vi "写入内置参数.vi"(7 "量程参数读取":T3 {"阈值（高->低）" format="%#.6g"; "阈值（低->高）" format="%#.6g"; "下限" format="%#.6g"; "上限" format="%#.6g"}, 8 "error in (no error)":errorcluster, 9 "float":T2 {"偏心轮校准参数" format="%#.6g"}, 10 "外设配置":T1 {"是否存在液位检测板" items=["否", "是"]; "阀数量" items=["9通"=9, "12通"=12]; "泵类型" items=["TECAN", "润泽"]}, 11 "MB session in":refnum<class "MB_Master.lvclass">) -> (0 "error out":errorcluster, 3 "MB session out":refnum<class "MB_Master.lvclass">)   [LabVIEW 2016, in "斯坦道CODMn新电路板.lvlib"]
uses:
  <vilib>/Plasmionique/MB Master/MB_Master/MB_Master.lvclass
  <vilib>/Plasmionique/MB Master/MB_Master_Serial/MB_Master_Serial.lvclass
  D:/Program Files (x86)/National Instruments/LabVIEW 2016/vi.lib/Plasmionique/MB Master/MB_Master/MB_Master.lvclass
  <vilib>/Plasmionique/MB Master/MB Master.lvlib
panel:
  in  "VISA Resource":refnum<visa-resource-name>
  in  "引用选择":enum16{"MB引用", "自建引用"}(ring)
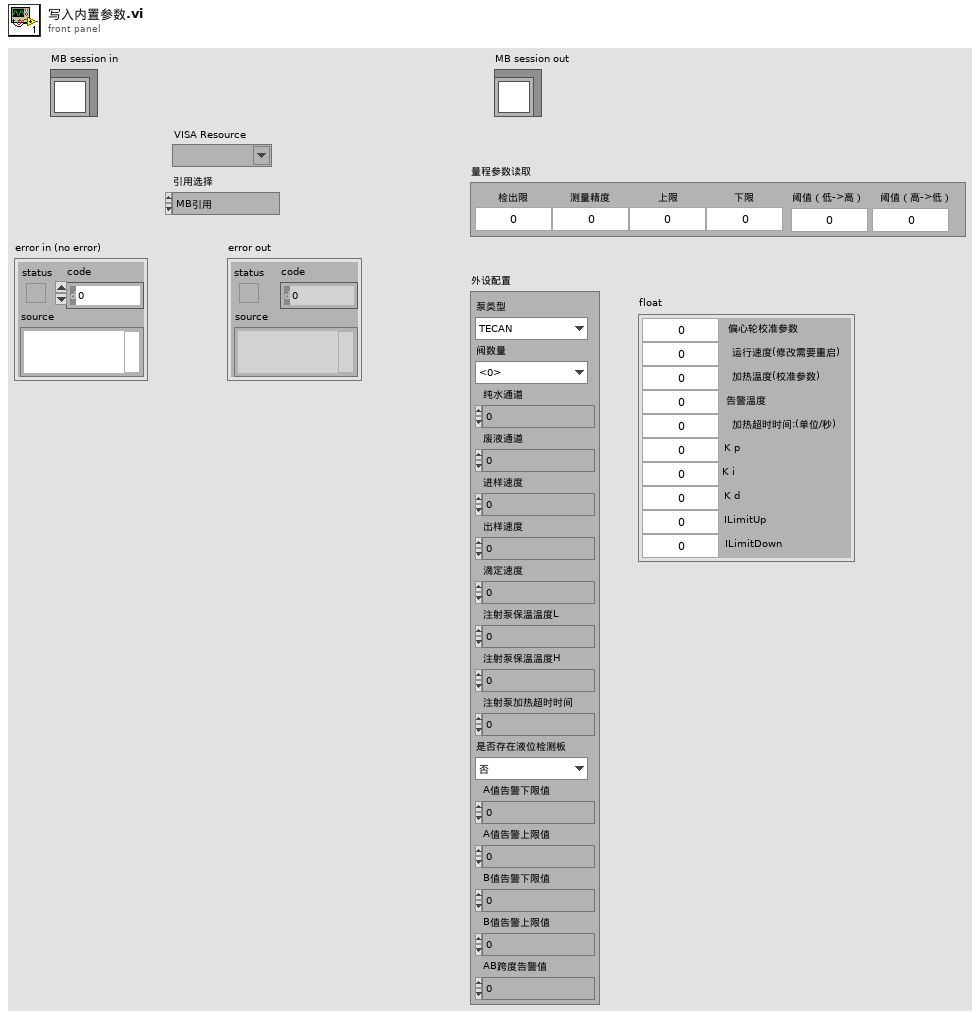
[diagram p1: front panel]
types:
  T1 = cluster{"泵类型":u8, "阀数量":u8, "纯水通道":u8, "废液通道":u8, "进样速度":u16, "出样速度":u16, "滴定速度":u16, "注射泵保温温度L":u8, "注射泵保温温度H":u8, "注射泵加热超时时间":u16, "是否存在液位检测板":u16, "A值告警下限值":u16, "A值告警上限值":u16, "B值告警下限值":u16, "B值告警上限值":u16, "AB跨度告警值":u16}
  T2 = cluster{"偏心轮校准参数":dbl, "运行速度(修改需要重启)":u16, "加热温度(校准参数) ":dbl, "告警温度":dbl, "加热超时时间:(单位/秒)":dbl, "K p":dbl, "K i":dbl, "K d":dbl, "ILimitUp":dbl, "ILimitDown":dbl}
  T3 = cluster{"检出限":dbl, "测量精度":dbl, "上限":dbl, "下限":dbl, "阈值（低->高）":dbl, "阈值（高->低）":dbl}
  T4 = cluster{"baud rate (bps)":u32, "stop bits":u16, "parity":u16, "flow control":u16, "timeout":u32, "retries":i32}
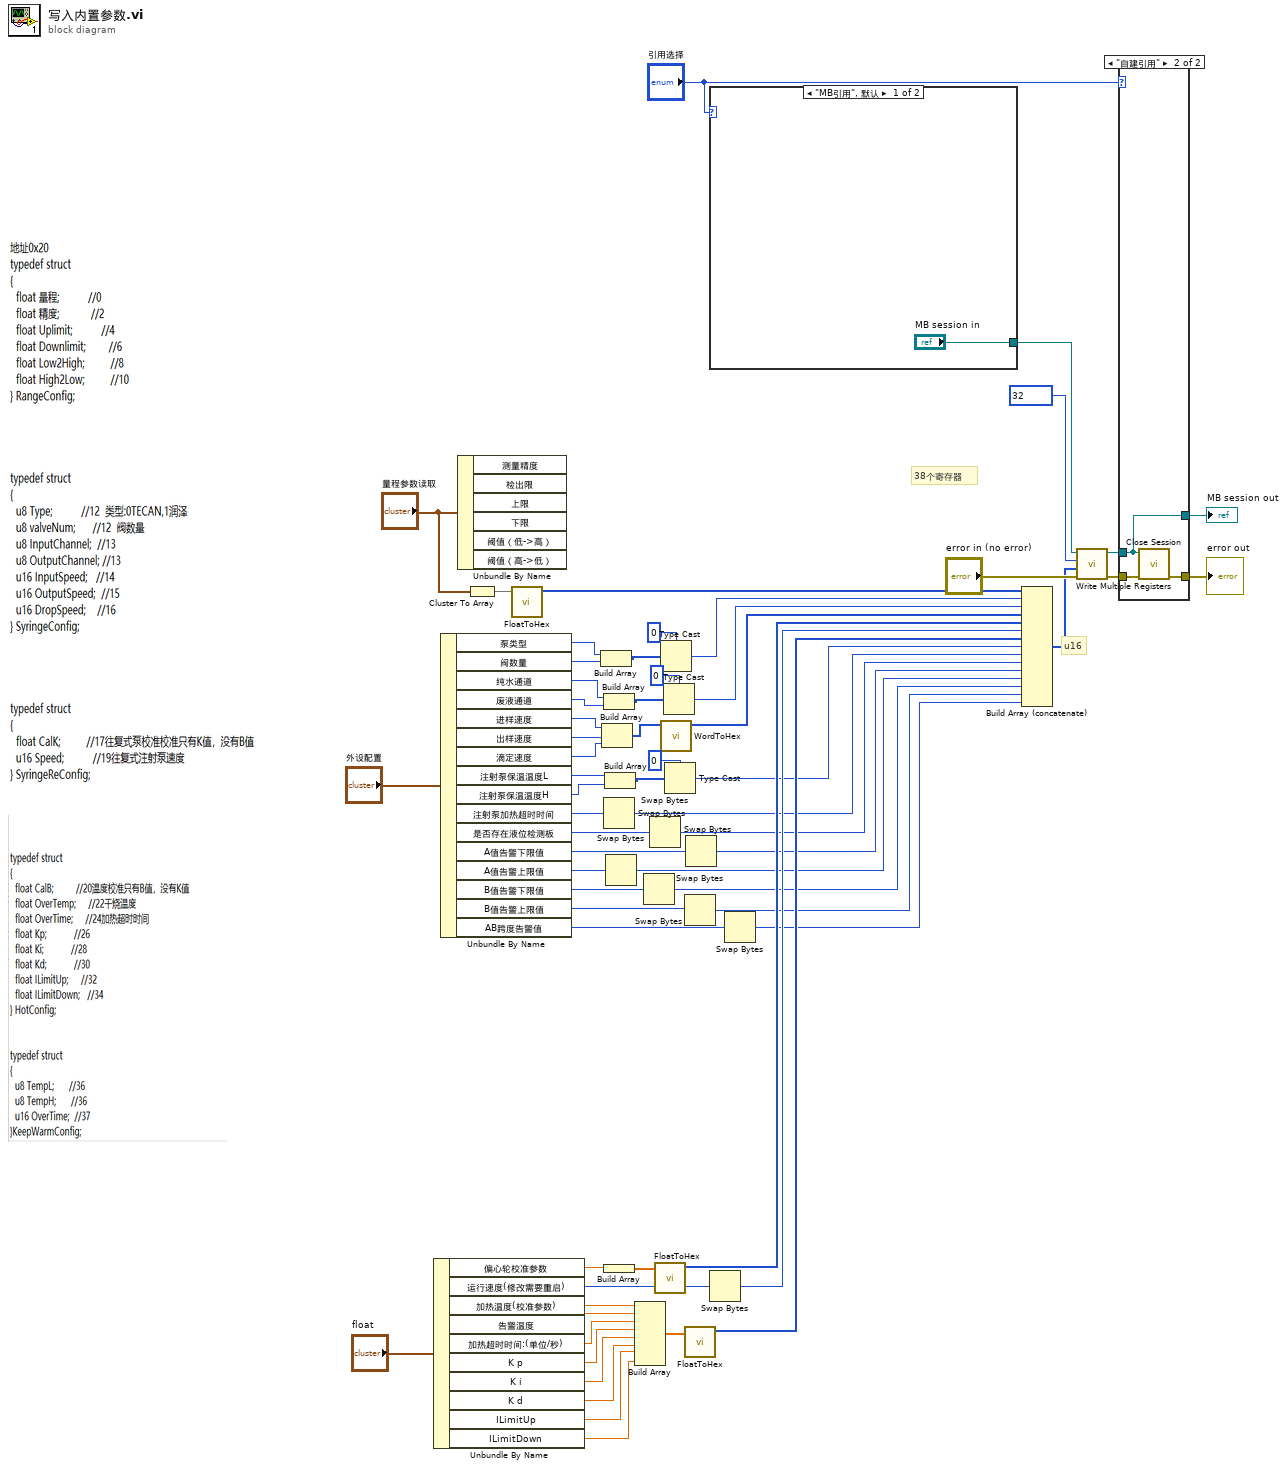
[diagram p0: block diagram]
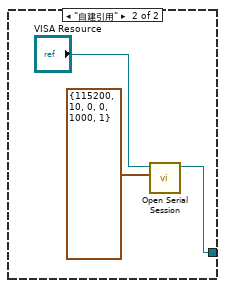
[diagram p3: hidden frame]
diagram:
  # "38个寄存器"
  # "u16"
  n1 = Unbundle By Name("float") -> ("偏心轮校准参数"=w40:dbl, "运行速度(修改需要重启)"=w17:u16, "加热温度(校准参数)"=w37:dbl, "告警温度"=w36:dbl, "加热超时时间:(单位/秒)"=w35:dbl, "K p"=w34:dbl, "K i"=w33:dbl, "K d"=w32:dbl, "ILimitUp"=w31:dbl, "ILimitDown"=w30:dbl)
  n2 = Unbundle By Name("外设配置") -> ("泵类型"=w52:u8, "阀数量"=w51:u8, "纯水通道"=w45:u8, "废液通道"=w44:u8, "进样速度"=w23:u16, "出样速度"=w22:u16, "滴定速度"=w21:u16, "注射泵保温温度L"=w26:u8, "注射泵保温温度H"=w25:u8, "注射泵加热超时时间"=w24:u16, "是否存在液位检测板"=w12:u16, "A值告警下限值"=w10:u16, "A值告警上限值"=w9:u16, "B值告警下限值"=w8:u16, "B值告警上限值"=w7:u16, "AB跨度告警值"=w6:u16)
  n3 = Unbundle By Name("量程参数读取") -> ()  [unwired: 6 out]
  n4 = Cluster To Array(cluster="量程参数读取") -> (array=w54:dbl[])
  n5 = call "FloatToHex.vi"("浮点数"=w54) -> ("DCBA整形输出"=w53:u16[])  [unwired: 10 in]
  n6 = Build Array(w52, w51) -> (w48:u8[])
  n7 = Build Array(w23, w22, w21) -> (w20:u16[])
  n8 = Build Array(w45, w44) -> (w47:u8[])
  n9 = Swap Bytes(anything=w24) -> (byte swapped=w13:u16)
  n10 = Build Array(w40) -> (w39:dbl[])
  n11 = Build Array(w26, w25) -> (w28:u8[])
  n12 = Swap Bytes(anything=w9) -> (byte swapped=w4:u16)
  n13 = Build Array(w37, w36, w35, w34, w33, w32, w31, w30) -> (w29:dbl[])
  n14 = Swap Bytes(anything=w8) -> (byte swapped=w3:u16)
  n15 = Swap Bytes(anything=w12) -> (byte swapped=w11:u16)
  n16 = call "FloatToHex.vi"("浮点数"=w39) -> ("DCBA整形输出"=w18:u16[])  [unwired: 10 in]
  n17 = Type Cast(type=u16 0, x=w48) -> (*(type *) &x=w42:u16)
  n18 = call "WordToHex.vi"("WORD"=w20) -> ("数组"=w19:u16[])  [unwired: 10 in]
  n19 = Type Cast(type=u16 0, x=w47) -> (*(type *) &x=w41:u16)
  n20 = Type Cast(type=u16 0, x=w28) -> (*(type *) &x=w14:u16)
  n21 = Swap Bytes(anything=w7) -> (byte swapped=w2:u16)
  n22 = call "FloatToHex.vi"("浮点数"=w29) -> ("DCBA整形输出"=w15:u16[])  [unwired: 10 in]
  n23 = Swap Bytes(anything=w10) -> (byte swapped=w5:u16)
  n24 = case shown="\"MB引用\", 默认" "引用选择" {
    tunnel: ["MB session in" w67] -> w61
    frame "MB引用", Default {
    }
    frame "自建引用" {
      n25 = call <vilib>:"Open Serial Session.vi"("Serial Config"=T4 {"baud rate (bps)"=115200, "stop bits"=10, "parity"=0, "flow control"=0, "timeout"=1000, "retries"=1}, "VISA Resource"="VISA Resource") -> ("MB_Serial session"=w67:refnum<class "MB_Master_Serial.lvclass">)  [unwired: 8 in, 1 out]
    }
  }
  n26 = Swap Bytes(anything=w17) -> (byte swapped=w16:u16)
  n27 = Swap Bytes(anything=w6) -> (byte swapped=w1:u16)
  n28 = Build Array (concatenate)(w53, w42, w41, w19, w18, w16, w15, w14, w13, w11, w5, w4, w3, w2, w1) -> (w43:u16[])
  n29 = call <vilib>:"Write Multiple Registers.vi"("error in (no error)"="error in (no error)", "values"=w43, "starting address"=u16 32, "MB session in"=w61) -> ("error out"=w58:errorcluster, "MB session out"=w60:refnum<class "MB_Master.lvclass">)  [unwired: 6 in]
  n30 = case shown="\"自建引用\"" "引用选择" {
    tunnel: w60 -> [w68 w70]
    tunnel: w58 -> [w69 w72]
    tunnel: [w69 w71] -> w57
    tunnel: [w68 w70] -> w56
    frame "MB引用", Default {
    }
    frame "自建引用" {
      n31 = call-dynamic "Close Session.vi"("error in (no error)"=w72, "MB session in"=w70) -> ("error out"=w71:errorcluster)  [unwired: 9 in]
    }
  }
  "MB session out" <- w56
  "error out" <- w57
